vi "DWE Popup Start.vi"() -> (0 "Date Laundry.NET\nstarted (MM_DD) 2":string, 1 "Folder to store data sets 2":path, 2 "End time save 2":string, 3 "Start time save 2":string, 4 "# of Files 2":i32, 6 "File directory 2":path)   [LabVIEW 2014]
doc: "Popup window for DWE program. User must provide information."
panel:
  in  "File directory":path
  in  "Done":bool
  in  "# of Files":i32=10
  in  "Date Laundry.NET\nstarted (MM_DD)":string
  in  "Folder to store data sets":path
  in  "Save data end time":string
  in  "Save data start time":string
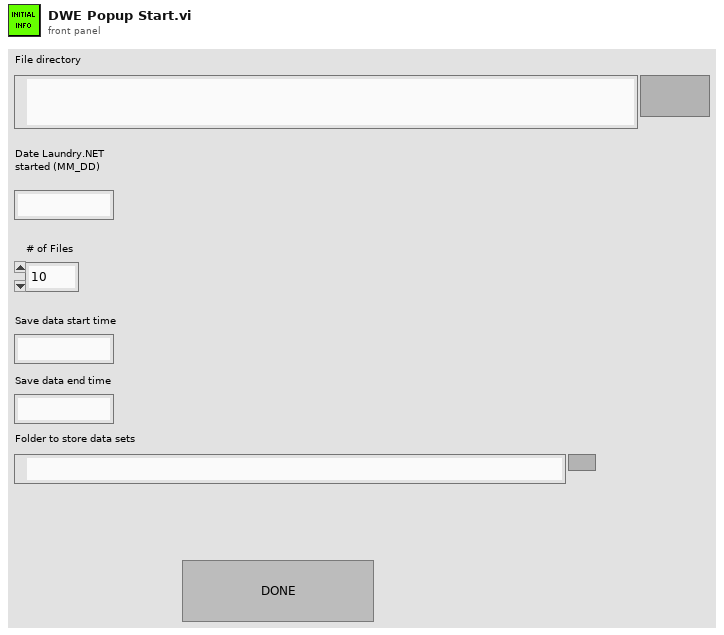
[diagram p1: front panel]
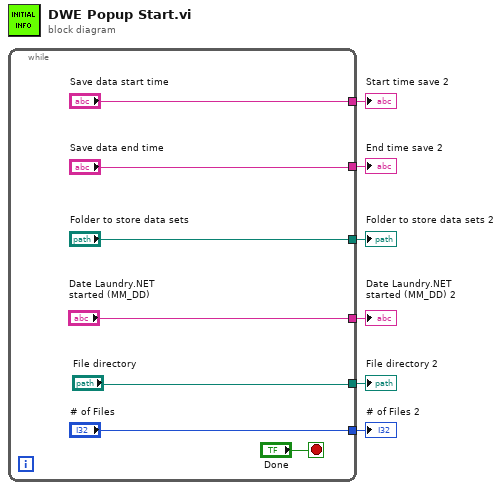
[diagram p0: block diagram]
diagram:
  n1 = while {
    tunnel: ["Save data start time"] -> w6
    tunnel: ["Save data end time"] -> w5
    tunnel: ["Folder to store data sets"] -> w4
    tunnel: ["Date Laundry.NET\nstarted (MM_DD)"] -> w3
    tunnel: ["File directory"] -> w1
    tunnel: ["# of Files"] -> w2
    stop <- "Done" stop-if-true
  }
  "Start time save 2" <- w6
  "End time save 2" <- w5
  "Folder to store data sets 2" <- w4
  "Date Laundry.NET\nstarted (MM_DD) 2" <- w3
  "# of Files 2" <- w2
  "File directory 2" <- w1
